vi "Excel Get References.vi"(8 "error in (no error)":errorcluster, 11 "npoiDocument in":refnum<class "npoiDocument.lvclass">) -> (0 "error out":errorcluster, 1 "Current Worksheet.Ref":refnum<k24>, 2 "Workbook.Ref":refnum<k24>, 3 "npoiDocument out":refnum<class "npoiDocument.lvclass">)   [LabVIEW 2017, in "NPOI_Document.lvlib" / "npoiDocument.lvclass"]
uses:
  npoiDocument.lvclass
  C:/Users/Neo/Desktop/Dev_Tools_BR/LabVIEW_NPOI/src/lib/NPOI 2.1.1/NPOI.dll
  lib/NPOI 2.1.1/NPOI.dll
  Excel_Specific/workbook/workbook.lvclass
  C:/Users/Neo/Desktop/Dev_Tools_BR/LabVIEW_NPOI/src/LabVIEW NPOI/NPOI_Document/npoiDocument/npoiDocument.lvclass
  Excel_Specific/workbook/workbook.lvclass/workbook.ctl
  Excel_Specific/workbook/Get Workbook.Ref.vi
  Excel_Specific/workbook/Get Active Worksheet Reference.vi
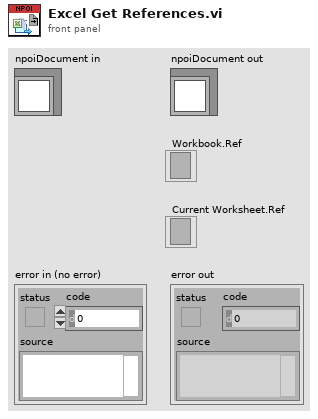
[diagram p1: front panel]
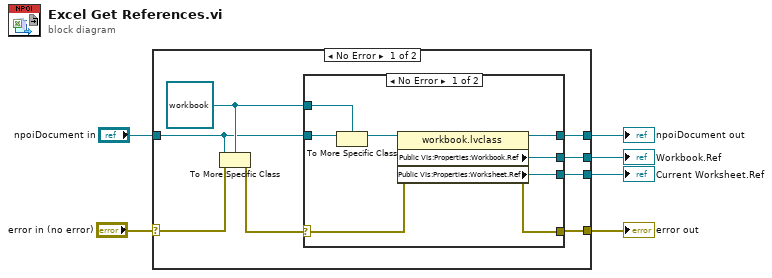
[diagram p0: block diagram]
diagram:
  n1 = case shown="No Error" "error in (no error)" {
    selector: "error in (no error)" -> [w12 w26]
    tunnel: [w11 w26] -> w5
    tunnel: [w14 w25] -> w3
    tunnel: "npoiDocument in" -> [w9 w25]
    tunnel: [w8 _] -> w2
    tunnel: [w7 _] -> w1
    frame No Error {
      w10 = refnum<class "workbook.lvclass"> refnum ("Excel_Specific.lvlib:workbook.lvclass")
      n2 = To More Specific Class(target class=w10, reference=w9, error in=w12) -> (error out=w13:errorcluster)  [unwired: 1 out]
      n3 = case shown="No Error" w13 {
        selector: w13 -> [w21 w24]
        tunnel: [w22 w23] -> w14
        tunnel: [w20 w24] -> w11
        tunnel: w10 -> [w19 _]
        tunnel: w9 -> [w18 w23]
        tunnel: [w16 _] -> w8
        tunnel: [w15 _] -> w7
        frame No Error {
          n4 = To More Specific Class(target class=w19, reference=w18) -> (specific class reference=w17:refnum<class "workbook.lvclass">)  [unwired: 1 in, 1 out]
          n5 = property class="workbook.lvclass"(reference=w17, error in=w21) -> (reference out=w22:refnum<class "workbook.lvclass">, error out=w20:errorcluster, "Public VIs:Properties:Workbook.Ref"=w16:refnum<k24>, "Public VIs:Properties:Worksheet.Ref"=w15:refnum<k24>)
        }
        frame Error {
        }
      }
    }
    frame Error {
    }
  }
  "error out" <- w5
  "npoiDocument out" <- w3
  "Workbook.Ref" <- w2
  "Current Worksheet.Ref" <- w1
